vi "createString.vi"(8 "error in (no error)":errorcluster, 10 "String":string, 11 "IString in":refnum<class "IString.lvclass">) -> (0 "error out":errorcluster, 3 "IString out":refnum<class "IString.lvclass">)   [LabVIEW 2022 SP3, in "openDAQ.lvlib" / "daqCoreTypes.lvlib" / "IString.lvclass"]
uses:
  <instrlib>/openDAQ/Public/Classes/daqCoreTypes/IString/IString.lvclass
  C:/Program Files (x86)/National Instruments/LabVIEW 2022/instr.lib/openDAQ/Public/Classes/IBaseObject/IBaseObject.lvclass
  <instrlib>/openDAQ/Public/Classes/IBaseObject/IBaseObject.lvclass/IBaseObject.ctl
  <instrlib>/openDAQ/Public/Classes/IBaseObject/Accessor/Read reference.vi
  <instrlib>/openDAQ/Public/Classes/IBaseObject/Accessor/Write reference.vi
  <instrlib>/openDAQ/Binaries/Windows/x86/copendaq32.dll
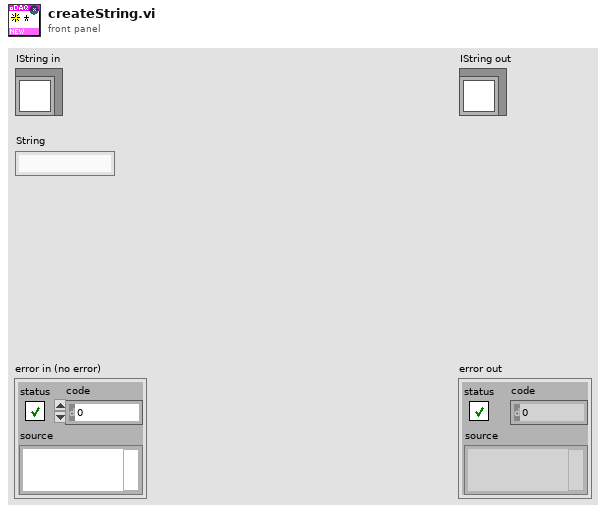
[diagram p1: front panel]
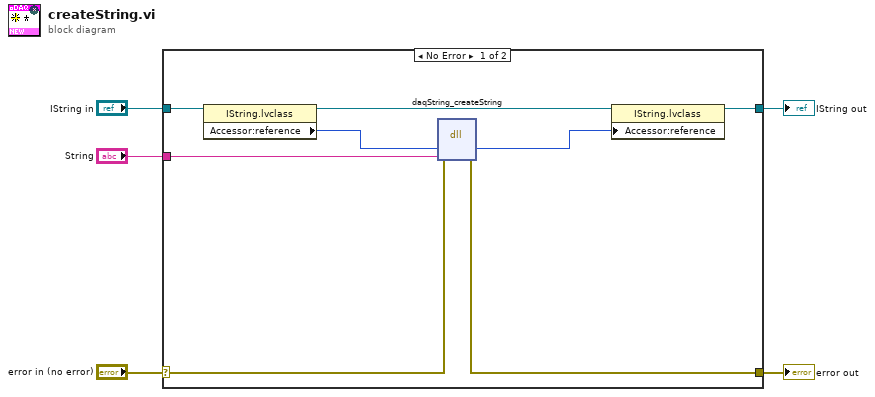
[diagram p0: block diagram]
diagram:
  n1 = case shown="No Error" "error in (no error)" {
    selector: "error in (no error)" -> [w12 w15]
    tunnel: [w11 w15] -> w4
    tunnel: [w7 w14] -> w2
    tunnel: "IString in" -> [w10 w14]
    tunnel: "String" -> [w13 _]
    frame No Error {
      n2 = property class="IString.lvclass"(reference=w10) -> (reference out=w8:refnum<class "IString.lvclass">, "Accessor:reference"=w9:i64)  [unwired: 1 in, 1 out]
      n3 = dll-call lib="C:/Program Files (x86)/National Instruments/LabVIEW 2022/instr.lib/openDAQ/Binaries/Windows/x86/copendaq*.*" fn="daqString_createString"(error in=w12, "daqString"=w9, "string"=w13) -> (error out=w11:errorcluster, "daqString"=w6:i64)  [unwired: 4 in, 1 out]
      n4 = property class="IString.lvclass"(reference=w8, "Accessor:reference"=w6) -> (reference out=w7:refnum<class "IString.lvclass">)  [unwired: 1 in, 1 out]
    }
    frame Error {
    }
  }
  "error out" <- w4
  "IString out" <- w2
